vi "GetDataForExcel.ReadPatientData_new.vi"(8 "error in":errorcluster, 11 "Path":path) -> (0 "error out":errorcluster, 3 "output cluster":T1)   [LabVIEW 2013, in "main.lvlib"]
uses:
  main.lvlib
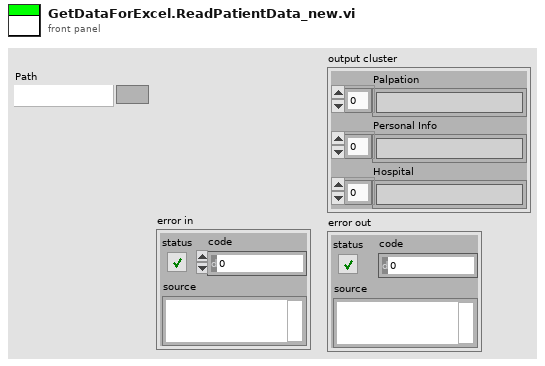
[diagram p1: front panel]
types:
  T1 = cluster{"Palpation":string[], "Personal Info":string[], "Hospital":string[]}
  T2 = cluster{"id":string, "name":string, "operator":string, "doctor":string, "comment":string}
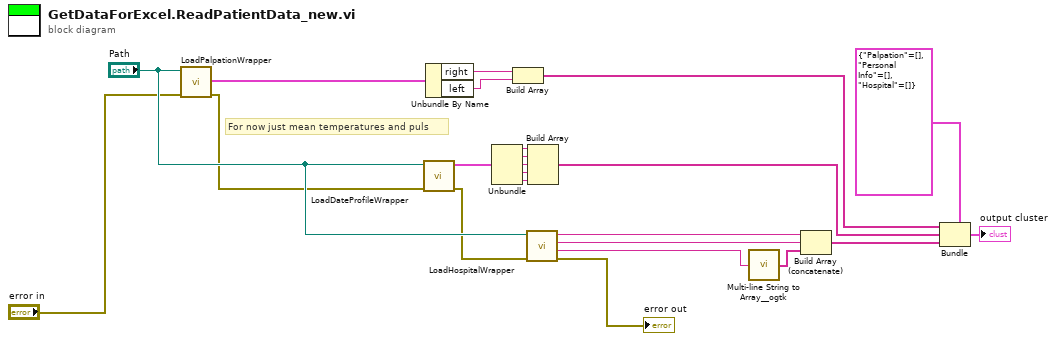
[diagram p0: block diagram]
diagram:
  # "For now just mean temperatures and puls"
  n1 = call "LoadPalpationWrapper.vi"("error in"="error in", "File dir"="Path") -> ("error out"=w3:errorcluster, "palpation"=w23:cluster{"right":string, "left":string})  [unwired: 8 in]
  n2 = call "LoadDateProfileWrapper.vi"("error in (no error)"=w3, "PatientDatePath"="Path") -> ("error out"=w2:errorcluster, "profile"=w16:T2)  [unwired: 8 in]
  n3 = Unbundle By Name(w23) -> ("right"=w22:string, "left"=w21:string)
  n4 = Unbundle(w16) -> ("id"=w11:string, "name"=w12:string, "operator"=w13:string, "doctor"=w14:string, "comment"=w15:string)
  n5 = Build Array(w22, w21) -> (w19:string[])
  n6 = call "LoadHospitalWrapper.vi"("error in (no error)"=w2, "PatientDatePath"="Path") -> ("error out"=→"error out":errorcluster, "Address"=w9:string, "Department"=w10:string, "Name"=w18:string)  [unwired: 6 in]
  n7 = Build Array(w11, w12, w13, w14, w15) -> (w6:string[])
  n8 = call <userlib>:"Multi-line String to Array__ogtk.vi"("string"=w9) -> ("lines"=w8:string[])
  n9 = Build Array (concatenate)(w18, w10, w8) -> (w7:string[])
  n10 = Bundle(cluster=T1 {"Palpation"=[], "Personal Info"=[], "Hospital"=[]} ("output cluster"), "Palpation"=w19, "Personal Info"=w6, "Hospital"=w7) -> (→"output cluster":T1)
